vi "change CAD coordinates.vi"() -> ()   [LabVIEW 2021]
uses:
  <vilib>/Analysis/coordinate.llb/2D Cartesian Coordinate Rotation (Scalar).vi
  <vilib>/Analysis/NI_AALPro.lvlib
panel:
  in  "Array 2":dbl[][](array[numeric])
  in  "Save to txt file":bool
  in  "Save picture":bool
  out "2D Picture":picture
  in  "Add delamination dots":bool
  in  "stop":bool
  in  "Rotate by angle":bool
  in  "theta (degrees)":dbl
  in  "Flip Y sign":bool
  in  "Flip X sign":bool
  in  "increase radius":bool
  in  "inc":dbl format="%#_13g"
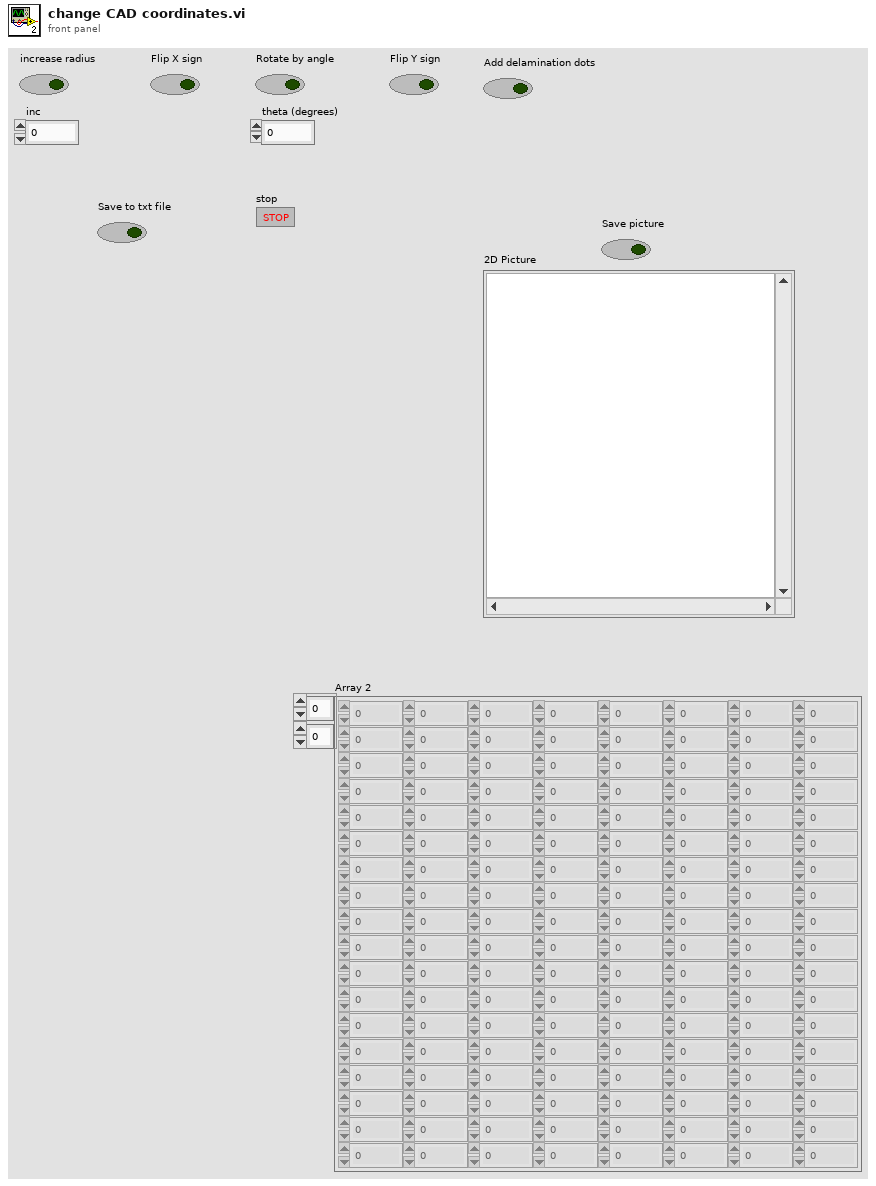
[diagram p1: front panel]
types:
  T1 = typedef "imagedata.ctl" = cluster{"image type":i32, "image depth":i32, "image":u8[], "mask":u8[], "colors":u32[], "Rectangle":cluster{"left":i16, "top":i16, "right":i16, "bottom":i16}}
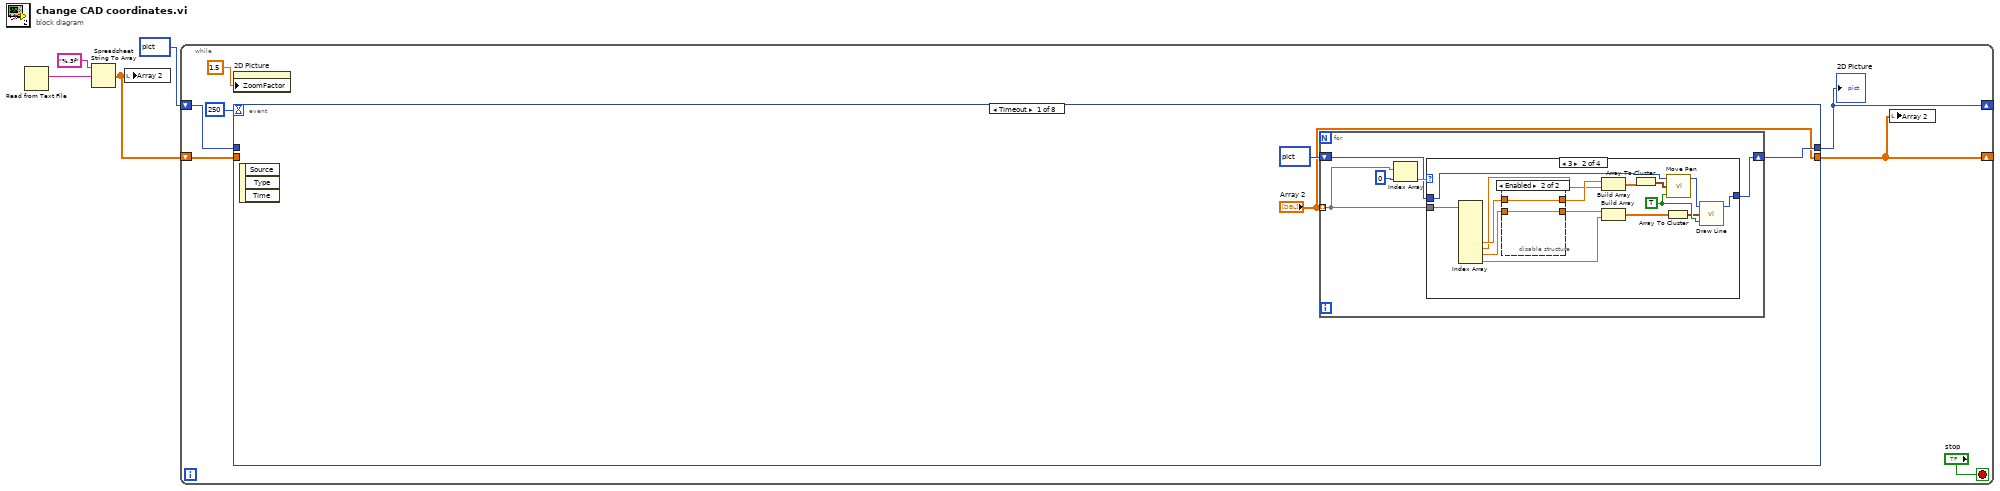
[diagram p0: block diagram]
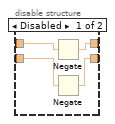
[diagram p3: hidden frame]
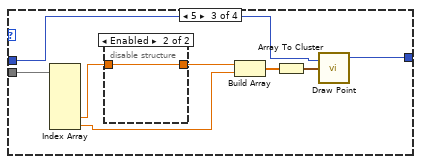
[diagram p4: hidden frame]
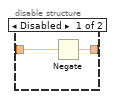
[diagram p5: hidden frame]
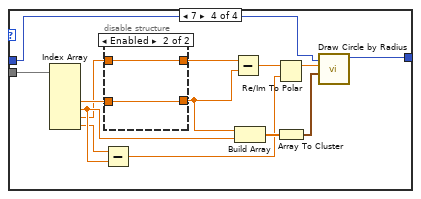
[diagram p6: hidden frame]
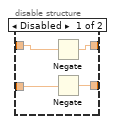
[diagram p7: hidden frame]
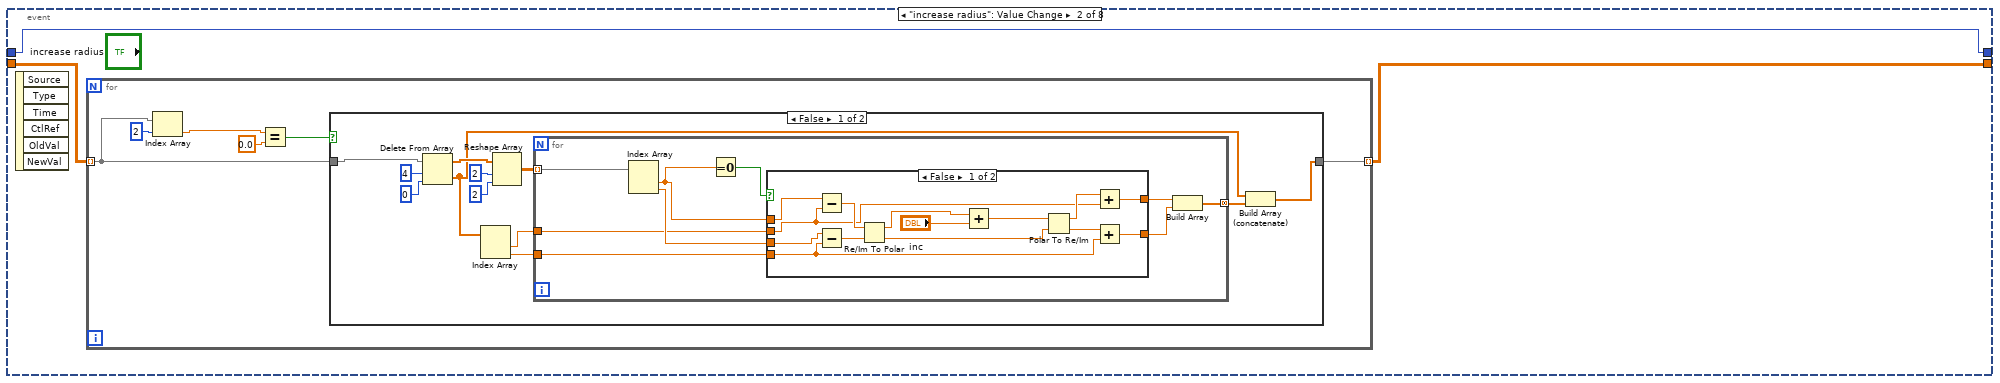
[diagram p8: hidden frame]
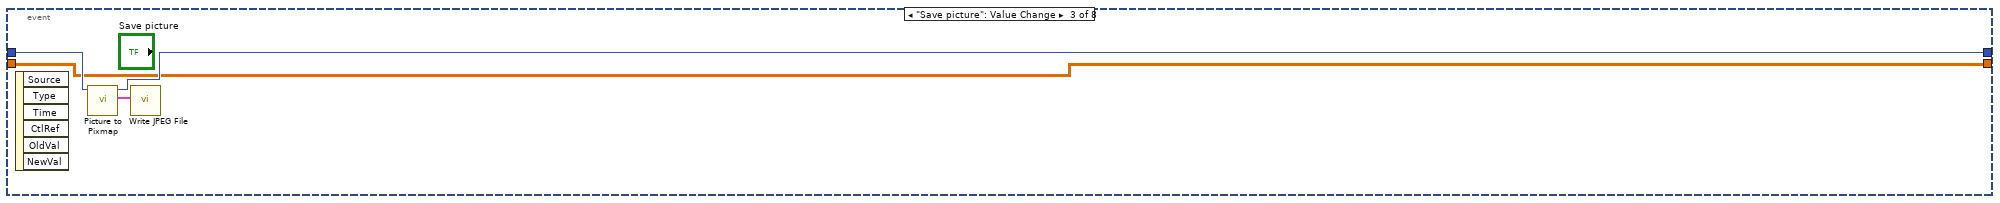
[diagram p11: hidden frame]
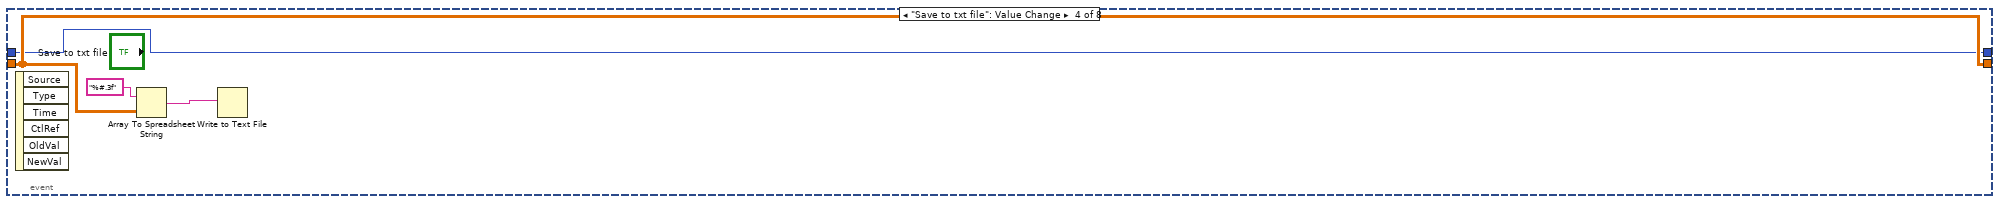
[diagram p12: hidden frame]
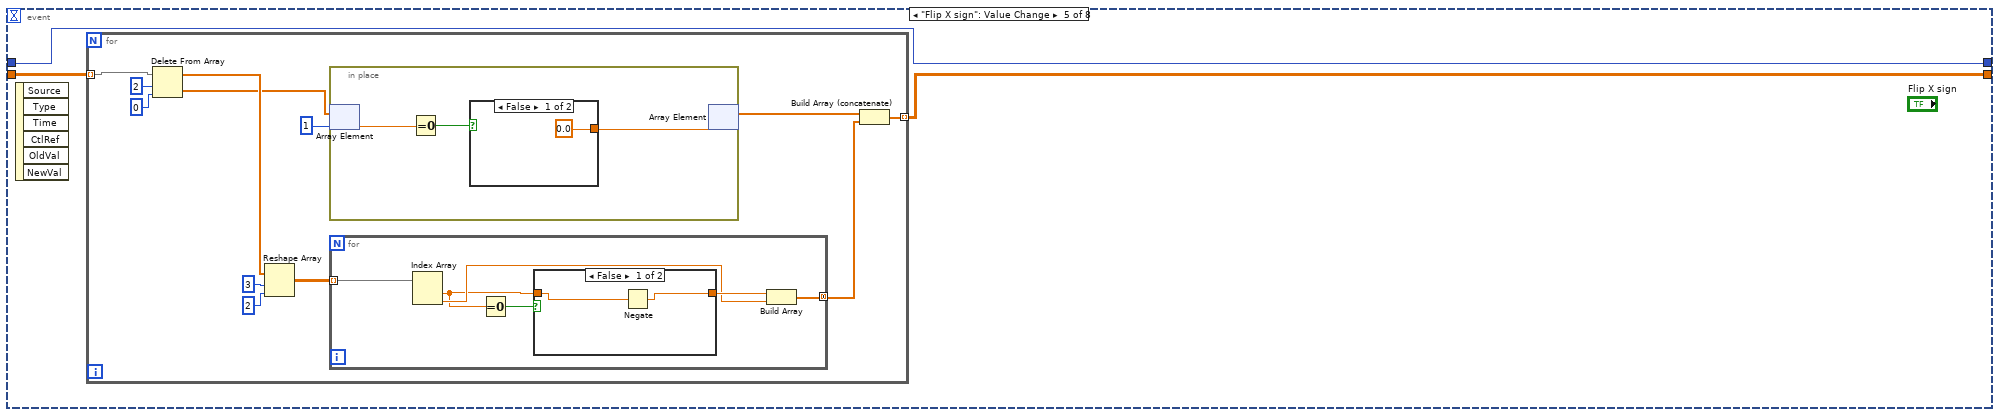
[diagram p13: hidden frame]
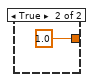
[diagram p14: hidden frame]
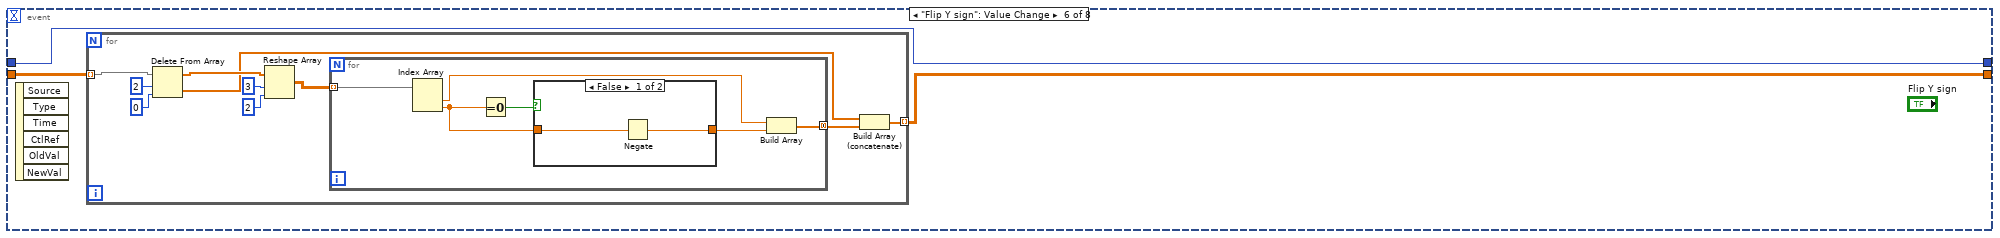
[diagram p16: hidden frame]
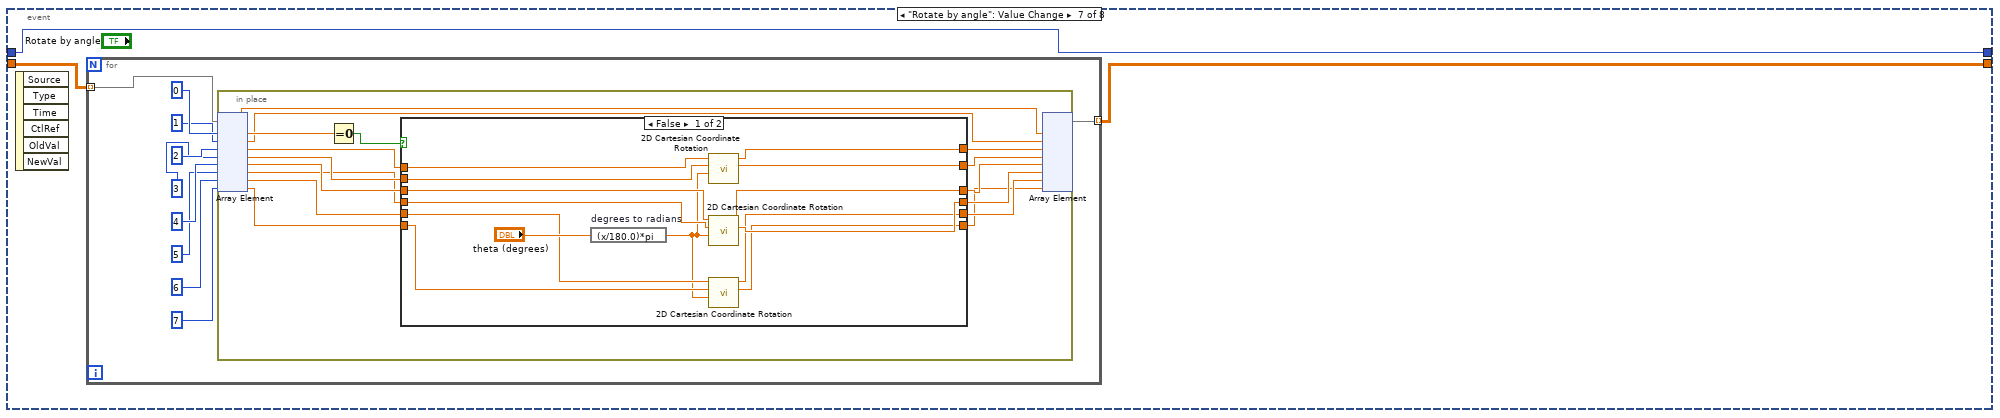
[diagram p18: hidden frame]
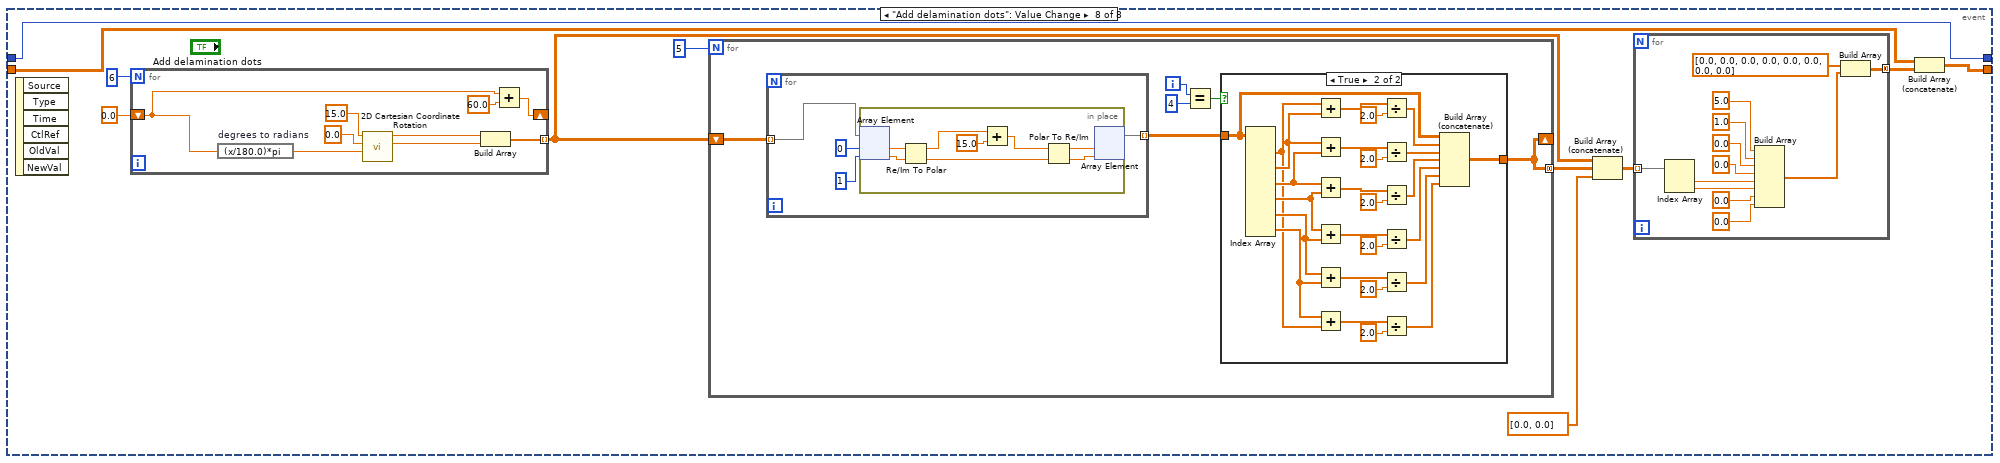
[diagram p20: hidden frame]
diagram:
  n1 = Read from Text File() -> (text=w4:string)  [unwired: 4 in, 3 out]
  n2 = Spreadsheet String To Array(format string="%.3f", spreadsheet string=w4) -> (array=w1:dbl[][])  [unwired: 2 in]
  n3 = local write "Array 2"(w1) -> ()
  n4 = while {
    shift-right: [w6] -> _
    shift-left: w1 -> [w9]
    shift-right: [w8] -> _
    shift-left: picture data[5B] ("picture") -> [w7]
    stop <- "stop" stop-if-true
    n5 = property on="2D Picture" class="Pict"("ZoomFactor"=sgl 1.5 ("Zoom Factor")) -> ()  [unwired: 2 in, 2 out]
    n6 = event shown="[0] Timeout" {
      selector: _ -> [_ _ _ _ _ _ _ _]
      dyn-events: _ -> [_ _ _ _ _ _ _ _]
      timeout: 250 -> [_ _ _ _ _ _ _ _]
      tunnel: w9 -> [_ w75 w120 w125 w130 w159 w181 w237]
      tunnel: ["Array 2" w74 w120 w125 w129 w158 w180 w228] -> w6
      tunnel: [w14 w73 w121 w124 w128 w157 w179 w227] -> w8
      tunnel: w7 -> [_ w73 w122 w124 w128 w157 w179 w227]
      event Timeout {
        n7 = event-data() -> ()  [unwired: 1 in, 3 out]
        n8 = for {
          tunnel: "Array 2" -> [w17] mode=indexing
          shift-right: [w15] -> w14
          shift-left: picture data[5B] ("picture") -> [w16]
          n9 = Index Array(array=w17, index=0) -> (element=w18:dbl)
          n10 = case shown="3" w18 {
            tunnel: w17 -> [_ w31 w47 w62]
            tunnel: w16 -> [w20 w33 w49 w66]
            tunnel: [w20 w35 w48 w65] -> w15
            frame 0, Default {
            }
            frame 3 {
              w32 = TRUE ("absolute coordinates?(T)")
              n11 = Index Array(array=w31) -> (element #5=w26:dbl, element #6=w24:dbl, element #7=w23:dbl, element #8=w21:dbl)  [unwired: 8 in, 4 out]
              n12 = disable-structure shown="Enabled" {
                disable-tunnel: w26 -> [w39 w41]
                disable-tunnel: [w38 w41] -> w25
                disable-tunnel: w23 -> [w37 w40]
                disable-tunnel: [w36 w40] -> w22
                frame Disabled {
                  n13 = Negate(x=w39) -> (-x=w38:dbl)
                  n14 = Negate(x=w37) -> (-x=w36:dbl)
                }
                frame Enabled {
                }
              }
              n15 = Build Array(w25, w24) -> (w30:dbl[])
              n16 = Build Array(w22, w21) -> (w28:dbl[])
              n17 = Array To Cluster(array=w30) -> (cluster=w29:cluster{"[0]":dbl, "[1]":dbl})
              n18 = Array To Cluster(array=w28) -> (cluster=w27:cluster{"[0]":dbl, "[1]":dbl})
              n19 = call <vilib>:"Move Pen.vi"("absolute coordinates?(T)"=w32, "new position"=w29, "picture"=w33) -> ("new picture"=w34:picture)  [unwired: 2 in]
              n20 = call <vilib>:"Draw Line.vi"("picture"=w34, "end point"=w27, "absolute coordinates?(T)"=w32) -> ("new picture"=w35:picture)  [unwired: 6 in]
            }
            frame 5 {
              n21 = Index Array(array=w47) -> (element #5=w44:dbl, element #6=w42:dbl)  [unwired: 6 in, 4 out]
              n22 = disable-structure shown="Enabled" {
                disable-tunnel: w44 -> [w51 w52]
                disable-tunnel: [w50 w52] -> w43
                frame Disabled {
                  n23 = Negate(x=w51) -> (-x=w50:dbl)
                }
                frame Enabled {
                }
              }
              n24 = Build Array(w43, w42) -> (w46:dbl[])
              n25 = Array To Cluster(array=w46) -> (cluster=w45:cluster{"[0]":dbl, "[1]":dbl})
              n26 = call <vilib>:"Draw Point.vi"("picture"=w49, "point(x,y)"=w45) -> ("new picture"=w48:picture)  [unwired: 7 in]
            }
            frame 7 {
              n27 = Index Array(array=w62) -> (element #3=w58:dbl, element #4=w56:dbl, element #5=w55:dbl, element #6=w53:dbl)  [unwired: 6 in, 2 out]
              n28 = Subtract(x=w53, y=w56) -> (x-y=w59:dbl)
              n29 = disable-structure shown="Enabled" {
                disable-tunnel: w58 -> [w70 w72]
                disable-tunnel: [w69 w72] -> w57
                disable-tunnel: w55 -> [w68 w71]
                disable-tunnel: [w67 w71] -> w54
                frame Disabled {
                  n30 = Negate(x=w68) -> (-x=w67:dbl)
                  n31 = Negate(x=w70) -> (-x=w69:dbl)
                }
                frame Enabled {
                }
              }
              n32 = Subtract(x=w54, y=w57) -> (x-y=w61:dbl)
              n33 = Build Array(w57, w56) -> (w64:dbl[])
              n34 = Re/Im To Polar(2:w59, 3:w61) -> (1:w60:dbl)  [unwired: 1 out]
              n35 = Array To Cluster(array=w64) -> (cluster=w63:cluster{"[0]":dbl, "[1]":dbl})
              n36 = call <vilib>:"Draw Circle by Radius.vi"("pixel center"=w63, "radius"=w60, "picture"=w66) -> ("new picture"=w65:picture)  [unwired: 8 in]
            }
          }
        }
      }
      event "increase radius": Value Change {
        n37 = event-data() -> ()  [unwired: 1 in, 6 out]
        n38 = for {
          tunnel: [w79] -> w74 mode=indexing
          tunnel: w75 -> [w78] mode=indexing
          n39 = Index Array(array=w78, index=2) -> (element=w76:dbl)
          n40 = Equal?(x=w76, y=0.0) -> (x = y?=w80:bool)
          n41 = case shown="False" w80 {
            tunnel: [w82 w119] -> w79
            tunnel: w78 -> [w88 w119]
            frame False {
              n42 = Delete From Array(array=w88, length=4, index=0) -> (deleted portion=w87:dbl[], array with subset deleted=w89:dbl[])
              n43 = Index Array(array=w87) -> (element #1=w85:dbl, element #2=w84:dbl)  [unwired: 2 in]
              n44 = Reshape Array(w89, 2 ("dimension size"), 2 ("dimension size")) -> (w86:dbl[][])
              n45 = for {
                tunnel: w86 -> [w102] mode=indexing
                tunnel: w85 -> [w100]
                tunnel: w84 -> [w96]
                tunnel: [w97] -> w83 mode=concatenating
                n46 = Index Array(array=w102) -> (element #1=w94:dbl, element #2=w101:dbl)  [unwired: 2 in]
                n47 = Equal To 0?(x=w94) -> (x = 0?=w95:bool)
                n48 = case shown="False" w95 {
                  tunnel: w94 -> [w116 w118]
                  tunnel: w101 -> [w114 w117]
                  tunnel: w100 -> [w107 _]
                  tunnel: [w106 w118] -> w99
                  tunnel: w96 -> [w104 _]
                  tunnel: [w103 w117] -> w98
                  frame False {
                    n49 = Subtract(x=w116, y=w107) -> (x-y=w115:dbl)
                    n50 = Subtract(x=w114, y=w104) -> (x-y=w113:dbl)
                    n51 = Re/Im To Polar(2:w113, 3:w115) -> (0:w110:dbl, 1:w112:dbl)
                    n52 = Add(x=w112, y="inc") -> (x+y=w109:dbl)
                    n53 = Polar To Re/Im(2:w110, 3:w109) -> (0:w105:dbl, 1:w108:dbl)
                    n54 = Add(x=w108, y=w107) -> (x+y=w106:dbl)
                    n55 = Add(x=w105, y=w104) -> (x+y=w103:dbl)
                  }
                  frame True {
                  }
                }
                n56 = Build Array(w99, w98) -> (w97:dbl[])
              }
              n57 = Build Array (concatenate)(w87, w83) -> (w82:dbl[])
            }
            frame True {
            }
          }
        }
      }
      event "Save picture": Value Change {
        n58 = event-data() -> ()  [unwired: 1 in, 6 out]
        n59 = call <vilib>:"Picture to Pixmap.vi"("picture"=w122) -> ("image data"=w123:T1, "new picture"=w121:picture)  [unwired: 9 in]
        n60 = call <vilib>:"Write JPEG File.vi"("image data"=w123) -> ()  [unwired: 9 in, 2 out]
      }
      event "Save to txt file": Value Change {
        n61 = event-data() -> ()  [unwired: 1 in, 6 out]
        n62 = Array To Spreadsheet String(array=w125, 3:"%#.3f" ("format string")) -> (spreadsheet string=w127:string)  [unwired: 1 in]
        n63 = Write to Text File(text=w127) -> ()  [unwired: 3 in, 3 out]
      }
      event "Flip X sign": Value Change {
        n64 = event-data() -> ()  [unwired: 1 in, 6 out]
        n65 = for {
          tunnel: w130 -> [w141] mode=indexing
          tunnel: [w142] -> w129 mode=indexing
          n66 = Delete From Array(array=w141, length=2, index=0) -> (deleted portion=w133:dbl[], array with subset deleted=w136:dbl[])
          n67 = Reshape Array(w136, 3 ("dimension size"), 2 ("dimension size")) -> (w135:dbl[][])
          n68 = in-place {
            n69 = in-place-array #1(w133, 1) -> (w144:dbl)
            n70 = Equal To 0?(x=w144) -> (x = 0?=w145:bool)
            n71 = case shown="False" w145 {
              tunnel: [0.0 1.0] -> w143
              frame False {
              }
              frame True {
              }
            }
            n72 = in-place-array #1(w143) -> (w132:dbl[])  [unwired: 1 out]
          }
          n73 = for {
            tunnel: w135 -> [w153] mode=indexing
            tunnel: [w150] -> w134 mode=concatenating
            n74 = Index Array(array=w153) -> (element #1=w148:dbl, element #2=w151:dbl)  [unwired: 2 in]
            n75 = Equal To 0?(x=w148) -> (x = 0?=w149:bool)
            n76 = case shown="False" w149 {
              tunnel: w148 -> [w155 w156]
              tunnel: [w154 w156] -> w152
              frame False {
                n77 = Negate(x=w155) -> (-x=w154:dbl)
              }
              frame True {
              }
            }
            n78 = Build Array(w152, w151) -> (w150:dbl[])
          }
          n79 = Build Array (concatenate)(w132, w134) -> (w142:dbl[])
        }
      }
      event "Flip Y sign": Value Change {
        n80 = event-data() -> ()  [unwired: 1 in, 6 out]
        n81 = for {
          tunnel: w159 -> [w168] mode=indexing
          tunnel: [w169] -> w158 mode=indexing
          n82 = Delete From Array(array=w168, length=2, index=0) -> (deleted portion=w161:dbl[], array with subset deleted=w163:dbl[])
          n83 = Reshape Array(w163, 3 ("dimension size"), 2 ("dimension size")) -> (w162:dbl[][])
          n84 = for {
            tunnel: w162 -> [w175] mode=indexing
            tunnel: [w174] -> w160 mode=concatenating
            n85 = Index Array(array=w175) -> (element #1=w171:dbl, element #2=w172:dbl)  [unwired: 2 in]
            n86 = Equal To 0?(x=w172) -> (x = 0?=w173:bool)
            n87 = case shown="False" w173 {
              tunnel: [w177 w178] -> w170
              tunnel: w172 -> [w176 w178]
              frame False {
                n88 = Negate(x=w176) -> (-x=w177:dbl)
              }
              frame True {
              }
            }
            n89 = Build Array(w171, w170) -> (w174:dbl[])
          }
          n90 = Build Array (concatenate)(w161, w160) -> (w169:dbl[])
        }
      }
      event "Rotate by angle": Value Change {
        n91 = event-data() -> ()  [unwired: 1 in, 6 out]
        n92 = for {
          tunnel: w181 -> [w191] mode=indexing
          tunnel: [w190] -> w180 mode=indexing
          n93 = in-place {
            n94 = in-place-array #2(w191, 0, 1, 2, 3, 4, 5, 6, 7) -> (w205:dbl, w204:dbl, w203:dbl, w200:dbl, w199:dbl, w196:dbl, w195:dbl, w192:dbl)
            n95 = Equal To 0?(x=w205) -> (x = 0?=w206:bool)
            n96 = case shown="False" w206 {
              tunnel: [w217 w226] -> w202
              tunnel: w203 -> [w220 w226]
              tunnel: w200 -> [w219 w225]
              tunnel: [w216 w225] -> w201
              tunnel: w199 -> [w215 w224]
              tunnel: [w213 w224] -> w198
              tunnel: [w212 w223] -> w197
              tunnel: w196 -> [w214 w223]
              tunnel: w195 -> [w209 w222]
              tunnel: [w211 w222] -> w194
              tunnel: [w210 w221] -> w193
              tunnel: w192 -> [w208 w221]
              frame False {
                n97 = expression code="(x/180.0)*pi" "degrees to radians"("theta (degrees)") -> (w207:dbl)
                n98 = call-poly <vilib>:"2D Cartesian Coordinate Rotation.vi"("theta"=w207, "y"=w219, "x"=w220) -> ("y out"=w216:dbl, "x out"=w217:dbl)  [unwired: 6 in, 1 out]
                n99 = call-poly <vilib>:"2D Cartesian Coordinate Rotation.vi"("theta"=w207, "y"=w214, "x"=w215) -> ("y out"=w212:dbl, "x out"=w213:dbl)  [unwired: 6 in, 1 out]
                n100 = call-poly <vilib>:"2D Cartesian Coordinate Rotation.vi"("theta"=w207, "y"=w208, "x"=w209) -> ("y out"=w210:dbl, "x out"=w211:dbl)  [unwired: 6 in, 1 out]
              }
              frame True {
              }
            }
            n101 = in-place-array #2(w205, w204, w202, w201, w198, w197, w194, w193) -> (w190:dbl[])  [unwired: 8 out]
          }
        }
      }
      event "Add delamination dots": Value Change {
        n102 = event-data() -> ()  [unwired: 1 in, 6 out]
        n103 = for {
          N: 6 -> [_]
          shift-right: [w301] -> _
          shift-left: 0.0 ("theta") -> [w297]
          tunnel: [w300] -> w234 mode=indexing
          n104 = expression code="(x/180.0)*pi" "degrees to radians"(w297) -> (w303:dbl)
          n105 = call-poly <vilib>:"2D Cartesian Coordinate Rotation.vi"("theta"=w303, "y"=0.0, "x"=15.0) -> ("y out"=w298:dbl, "x out"=w299:dbl)  [unwired: 6 in, 1 out]
          n106 = Build Array(w299, w298) -> (w300:dbl[])
          n107 = Add(x=w297, y=60.0) -> (x+y=w301:dbl)
        }
        n108 = for {
          N: 5 -> [_]
          shift-right: [w252] -> _
          shift-left: w234 -> [w255]
          tunnel: [w252] -> w233 mode=concatenating
          i -> [w251]
          n109 = for {
            tunnel: w255 -> [w286] mode=indexing
            tunnel: [w285] -> w253 mode=indexing
            n110 = in-place {
              n111 = in-place-array #3(w286, 0, 1) -> (w290:dbl, w289:dbl)
              n112 = Re/Im To Polar(2:w289, 3:w290) -> (0:w291:dbl, 1:w293:dbl)
              n113 = Add(x=w293, y=15.0) -> (x+y=w292:dbl)
              n114 = Polar To Re/Im(2:w291, 3:w292) -> (0:w287:dbl, 1:w288:dbl)
              n115 = in-place-array #3(w288, w287) -> (w285:dbl[])  [unwired: 2 out]
            }
          }
          n116 = Equal?(x=w251, y=4) -> (x = y?=w254:bool)
          n117 = case shown="True" w254 {
            tunnel: w253 -> [w256 w280]
            tunnel: [w256 w257] -> w252
            frame False {
            }
            frame True {
              n118 = Index Array(array=w280) -> (element #1=w259:dbl[], element #2=w277:dbl[], element #3=w272:dbl[], element #4=w268:dbl[], element #5=w264:dbl[], element #6=w260:dbl[])  [unwired: 12 in]
              n119 = Add(x=w259, y=w277) -> (x+y=w282:dbl[])
              n120 = Add(x=w277, y=w272) -> (x+y=w278:dbl[])
              n121 = Add(x=w272, y=w268) -> (x+y=w274:dbl[])
              n122 = Add(x=w268, y=w264) -> (x+y=w270:dbl[])
              n123 = Add(x=w264, y=w260) -> (x+y=w266:dbl[])
              n124 = Add(x=w260, y=w259) -> (x+y=w262:dbl[])
              n125 = Divide(x=w282, y=2.0) -> (x/y=w279:dbl[])
              n126 = Divide(x=w278, y=2.0) -> (x/y=w275:dbl[])
              n127 = Divide(x=w274, y=2.0) -> (x/y=w271:dbl[])
              n128 = Divide(x=w270, y=2.0) -> (x/y=w267:dbl[])
              n129 = Divide(x=w266, y=2.0) -> (x/y=w263:dbl[])
              n130 = Divide(x=w262, y=2.0) -> (x/y=w258:dbl[])
              n131 = Build Array (concatenate)(w280, w279, w275, w271, w267, w263, w258) -> (w257:dbl[][])
            }
          }
        }
        n132 = Build Array (concatenate)(w234, w233, dbl[] [0.0, 0.0] ("array")) -> (w231:dbl[][])
        n133 = for {
          tunnel: w231 -> [w245] mode=indexing
          tunnel: [w240] -> w229 mode=concatenating
          n134 = Index Array(array=w245) -> (element #1=w244:dbl, element #2=w243:dbl)  [unwired: 2 in]
          n135 = Build Array(5.0 ("element"), 1.0 ("element"), 0.0 ("element"), 0.0 ("element"), w244, w243, 0.0 ("element"), 0.0 ("element")) -> (w238:dbl[])
          n136 = Build Array(dbl[] [0.0, 0.0, 0.0, 0.0, 0.0, 0.0, 0.0, 0.0] ("array"), w238) -> (w240:dbl[][])
        }
        n137 = Build Array (concatenate)(w237, w229) -> (w228:dbl[][])
      }
    }
    "2D Picture" <- w8
    n138 = local write "Array 2"(w6) -> ()
  }
